vi "TDTSyn-Get Events Final.vi"(0 "State":T1, 5 "URL":string="http://localhost:24414", 11 "error in (no error)":errorcluster) -> (4 "Data out":T1, 8 "Events":dbl[][](array[numeric]), 10 "total ticks":i32, 14 "NumTicks":i32, 15 "error out":errorcluster)   [LabVIEW 2020]
uses:
  TDTSyn-State.ctl
panel:
  in  "Poll Interval (s)":dbl=2.0
  in  "Timeout (s)":dbl=10.0
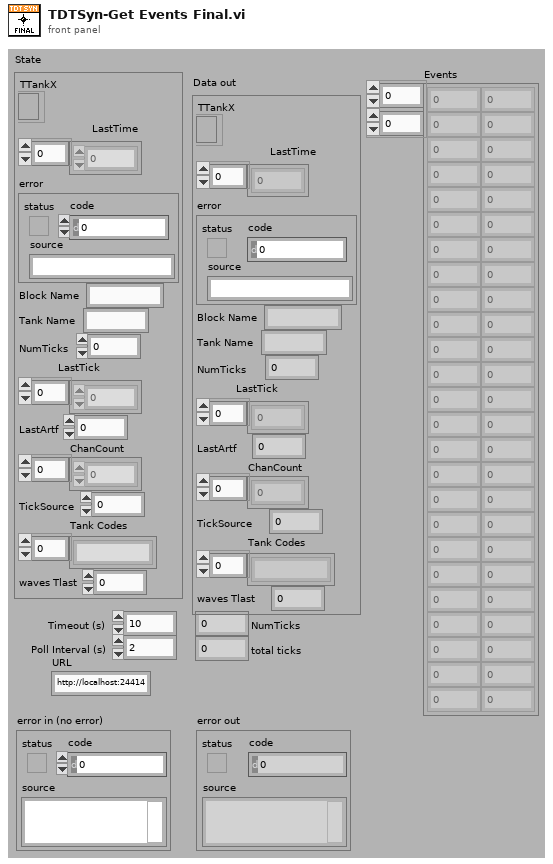
[diagram p1: front panel]
types:
  T1 = typedef "TDTSyn-State.ctl" = cluster{"TTankX":refnum<k7>, "LastTime":dbl[], "error":errorcluster, "Block Name":string, "Tank Name":string, "NumTicks":i32, "LastTick":dbl[], "LastArtf":dbl, "ChanCount":i32[], "TickSource":i32, "Tank Codes":string[], "waves Tlast":dbl}
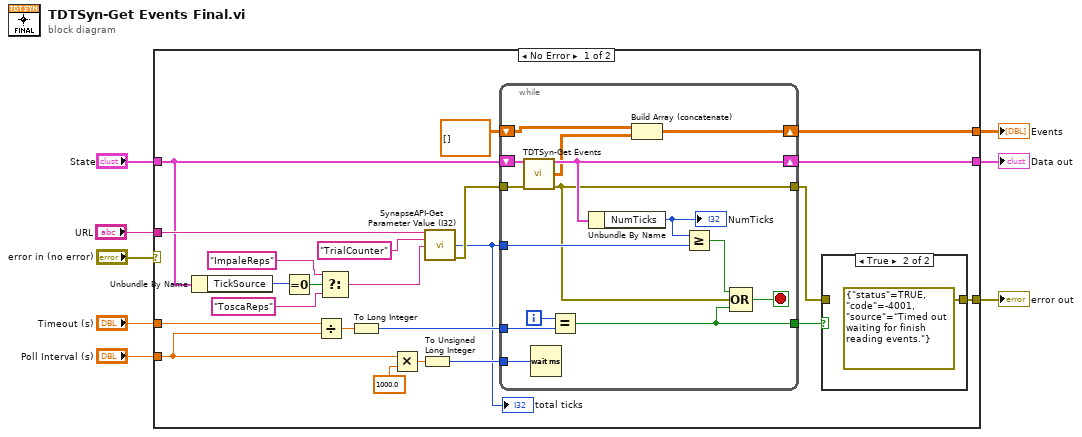
[diagram p0: block diagram]
diagram:
  n1 = case shown="No Error" "error in (no error)" {
    selector: "error in (no error)" -> [_ w50]
    tunnel: [w23 w50] -> w7
    tunnel: "State" -> [w14 w49]
    tunnel: "Timeout (s)" -> [w28 _]
    tunnel: "Poll Interval (s)" -> [w27 _]
    tunnel: [w21 w49] -> w3
    tunnel: [w20 _] -> w2
    tunnel: "URL" -> [w16 _]
    frame No Error {
      n2 = Unbundle By Name(w14) -> ("TickSource"=w13:i32)
      n3 = Equal To 0?(x=w13) -> (x = 0?=w12:bool)
      n4 = Divide(x=w28, y=w27) -> (x/y=w31:dbl)
      n5 = Select(t="ImpaleReps" ("Parameter"), s=w12, f="ToscaReps" ("Parameter")) -> (s? t:f=w10:string)
      n6 = To Long Integer(number=w31) -> (32bit integer=w25:i32)
      n7 = Multiply(x=w27, y=1000.0) -> (x*y=w30:dbl)
      n8 = To Unsigned Long Integer(number=w30) -> (unsigned 32bit integer=w26:u32)
      n9 = call "SynapseAPI-Get Parameter Value (I32).vi"("URL"=w16, "Gizmo"="TrialCounter", "Parameter"=w10) -> ("value"=w17:i32, "error out"=w18:errorcluster)  [unwired: 11 in]
      "total ticks" <- w17
      n10 = while {
        tunnel: w18 -> [w42]
        tunnel: w26 -> [w47]
        tunnel: w25 -> [w45]
        tunnel: [w43] -> w24
        tunnel: w17 -> [w39]
        shift-right: [w41] -> w21
        shift-left: w14 -> [w34]
        tunnel: [w35] -> w22
        shift-right: [w37] -> w20
        shift-left: dbl[][] [] -> [w36]
        i -> [w46]
        stop <- w48 stop-if-true
        n11 = call "TDTSyn-Get Events.vi"("State In"=w34, "error in (no error)"=w42) -> ("State Out"=w41:T1, "Events"=w38:dbl[][], "error out"=w35:errorcluster)  [unwired: 10 in, 1 out]
        n12 = Wait (ms)(milliseconds to wait=w47) -> ()  [unwired: 1 out]
        n13 = Equal?(x=w46, y=w45) -> (x = y?=w43:bool)
        n14 = Unbundle By Name(w41) -> ("NumTicks"=w40:i32)
        "NumTicks" <- w40
        n15 = Build Array (concatenate)(w36, w38) -> (w37:dbl[][])
        n16 = Greater Or Equal?(x=w40, y=w39) -> (x >= y?=w44:bool)
        n17 = Compound Arithmetic op=OR(w44, w35, w43) -> (w48:bool)
      }
      n18 = case shown="True" w24 {
        tunnel: [w32 errorcluster {"status"=TRUE, "code"=-4001, "source"="Timed out waiting for finish reading events."} ("error out")] -> w23
        tunnel: w22 -> [w32 _]
        frame False {
        }
        frame True {
        }
      }
    }
    frame Error {
    }
  }
  "error out" <- w7
  "Data out" <- w3
  "Events" <- w2
